vi "Unlock Mutex.vi"(8 "error in (no error)":errorcluster, 10 "Owner":string, 11 "Mutex In":T1) -> (0 "error out":errorcluster, 3 "Mutex Out":T1)   [LabVIEW 2021]
uses:
  <vilib>/myRIO/Common/Instrument Driver Framework/Utilities/typedefs/Reentrant Mutex.ctl
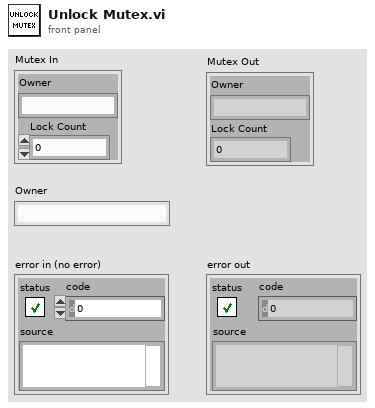
[diagram p1: front panel]
types:
  T1 = typedef "Reentrant Mutex.ctl" = cluster{"Owner":string, "Lock Count":u32}
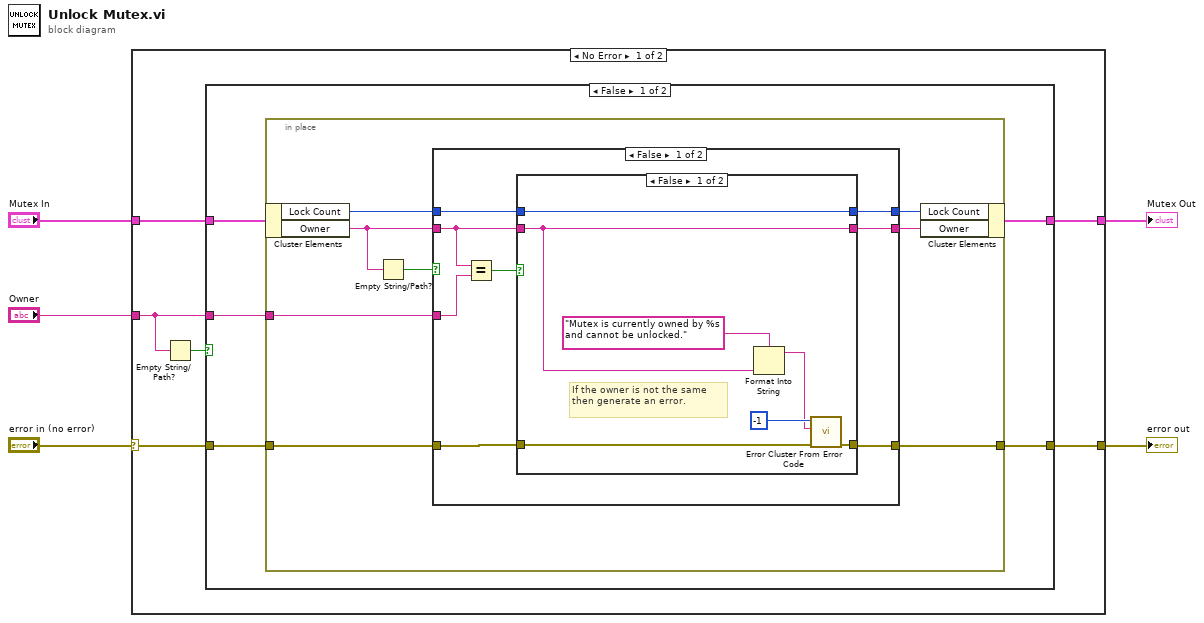
[diagram p0: block diagram]
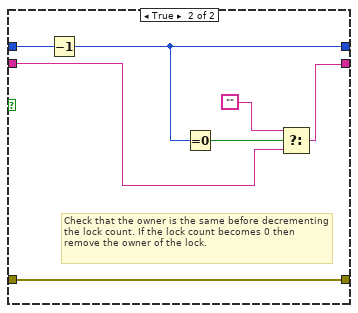
[diagram p2: hidden frame]
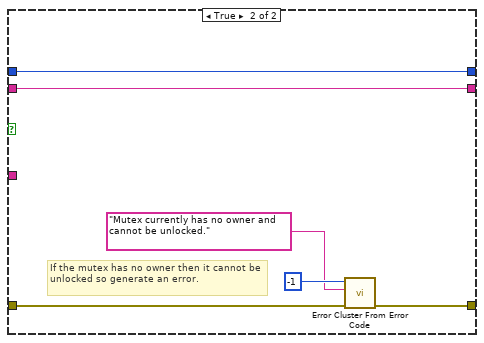
[diagram p3: hidden frame]
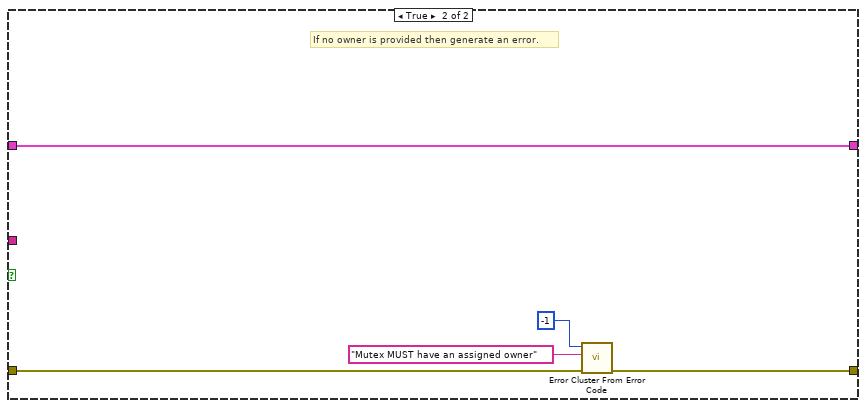
[diagram p4: hidden frame]
diagram:
  n1 = case shown="No Error" "error in (no error)" {
    selector: "error in (no error)" -> [w10 w59]
    tunnel: "Mutex In" -> [w8 w58]
    tunnel: "Owner" -> [w6 _]
    tunnel: [w9 w59] -> w2
    tunnel: [w7 w58] -> w1
    frame No Error {
      n2 = Empty String/Path?(string/path=w6) -> (empty?=w11:bool)
      n3 = case shown="False" w11 {
        tunnel: w10 -> [w16 w57]
        tunnel: [w14 w56] -> w9
        tunnel: w8 -> [w13 w53]
        tunnel: w6 -> [w15 _]
        tunnel: [w12 w53] -> w7
        frame False {
          n4 = in-place {
            in-place-border: w16 -> [w24]
            in-place-border: w15 -> [w23]
            in-place-border: [w22] -> w14
            n5 = in-place-cluster #1(w13) -> ("Lock Count"=w21:u32, "Owner"=w18:string)
            n6 = Empty String/Path?(string/path=w18) -> (empty?=w17:bool)
            n7 = case shown="False" w17 {
              tunnel: w24 -> [w32 w51]
              tunnel: w23 -> [w31 _]
              tunnel: [w30 w50] -> w22
              tunnel: w21 -> [w29 w48]
              tunnel: [w28 w48] -> w20
              tunnel: [w27 w47] -> w19
              tunnel: w18 -> [w26 w47]
              frame False {
                n8 = Equal?(x=w26, y=w31) -> (x = y?=w25:bool)
                n9 = case shown="False" w25 {
                  tunnel: w29 -> [w39 w46]
                  tunnel: [w39 w44] -> w28
                  tunnel: [w34 w40] -> w27
                  tunnel: w26 -> [w34 w42]
                  tunnel: w32 -> [w37 w45]
                  tunnel: [w36 w45] -> w30
                  frame False {
                    # "If the owner is not the same then generate an error."
                    n10 = Format Into String(format string="Mutex is currently owned by %s and cannot be unlocked." ("error message (\"\")"), w34) -> (resulting string=w35:string)  [unwired: 2 in, 1 out]
                    n11 = call <vilib>:"Error Cluster From Error Code.vi"("error in (no error)"=w37, "error message (\"\")"=w35, "error code (0)"=-1) -> ("error out"=w36:errorcluster)  [unwired: 6 in]
                  }
                  frame True {
                    # "Check that the owner is the same before decrementing the lock count. If the lock count becomes 0 then remove the owner of the lock."
                    n12 = Decrement(x=w46) -> (x-1=w44:u32)
                    n13 = Equal To 0?(x=w44) -> (x = 0?=w43:bool)
                    n14 = Select(t="", s=w43, f=w42) -> (s? t:f=w40:string)
                  }
                }
              }
              frame True {
                # "If the mutex has no owner then it cannot be unlocked so generate an error."
                n15 = call <vilib>:"Error Cluster From Error Code.vi"("error in (no error)"=w51, "error message (\"\")"="Mutex currently has no owner and cannot be unlocked." ("error message (\"\")"), "error code (0)"=-1) -> ("error out"=w50:errorcluster)  [unwired: 6 in]
              }
            }
            n16 = in-place-cluster #1("Lock Count"=w20, "Owner"=w19) -> (w12:T1)
          }
        }
        frame True {
          # "If no owner is provided then generate an error."
          n17 = call <vilib>:"Error Cluster From Error Code.vi"("error in (no error)"=w57, "error message (\"\")"="Mutex MUST have an assigned owner" ("error message (\"\")"), "error code (0)"=-1) -> ("error out"=w56:errorcluster)  [unwired: 6 in]
        }
      }
    }
    frame Error {
      # "There is an error coming in so there is nothing to be done."
    }
  }
  "Mutex Out" <- w1
  "error out" <- w2
